vi "writeFlash.vi"(1 "bytesToWrite":u32, 2 "offset":u32, 3 "buffer":u8[](array[numeric])) -> (0 "return type":i32)   [LabVIEW 2012]
uses:
  hidapi_32bits.dll
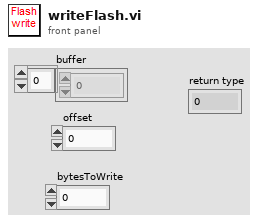
[diagram p1: front panel]
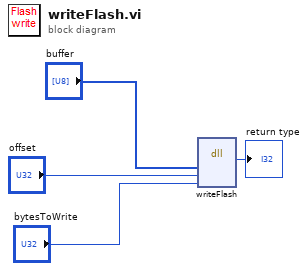
[diagram p0: block diagram]
diagram:
  n1 = dll-call lib="C:/All_Data/mikrocont/Project1/New_controller__Jan_2015/LabView_Aug_2015/hidapi_32bits.dll" fn="writeFlash"("buffer"="buffer", "offset"="offset", "bytesToWrite"="bytesToWrite") -> ("return type"=→"return type":i32)  [unwired: 6 in, 2 out]
